vi "Write millisecond timer value.vi"(8 "error in (no error)":errorcluster, 10 "millisecond timer value":u32, 11 "Wait Step in":refnum<class "Wait Step.lvclass">) -> (0 "error out":errorcluster, 3 "Wait Step out":refnum<class "Wait Step.lvclass">)   [LabVIEW 2015, in "Wait Step.lvclass"]
uses:
  Wait Step.lvclass
  Wait Step.lvclass/Wait Step.ctl
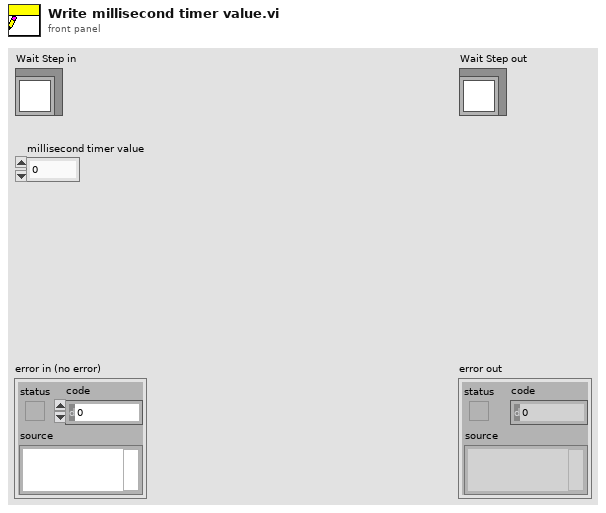
[diagram p1: front panel]
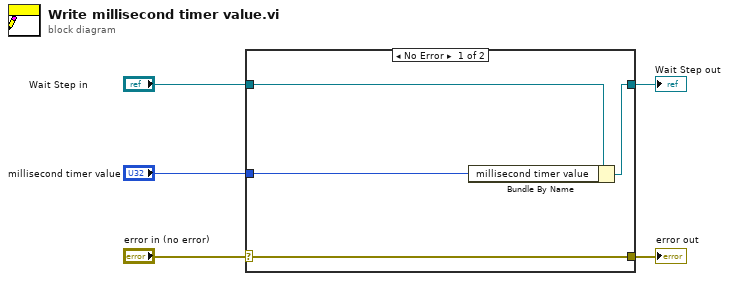
[diagram p0: block diagram]
diagram:
  n1 = case shown="No Error" "error in (no error)" {
    selector: "error in (no error)" -> [w9 w10]
    tunnel: [w9 w10] -> w4
    tunnel: [w7 w11] -> w2
    tunnel: "Wait Step in" -> [w8 w11]
    tunnel: "millisecond timer value" -> [w6 _]
    frame No Error {
      n2 = Bundle By Name(cluster=w8, "millisecond timer value"=w6) -> (w7:refnum<class "Wait Step.lvclass">)
    }
    frame Error {
    }
  }
  "error out" <- w4
  "Wait Step out" <- w2
